vi "Core-GetTicks.vi"(8 "error in (no error)":errorcluster, 11 "Engine in":refnum<class "Engine.lvclass">) -> (0 "error out":errorcluster, 3 "Engine out":refnum<class "Engine.lvclass">)   [LabVIEW 2024, in "GLF.lvlib" / "Engine.lvclass"]
uses:
  Engine.lvclass
  Engine.lvclass/Engine.ctl
  <vilib>/Saukko/LV SDL3/Sources/SDL3/Timer/Timer.lvlib
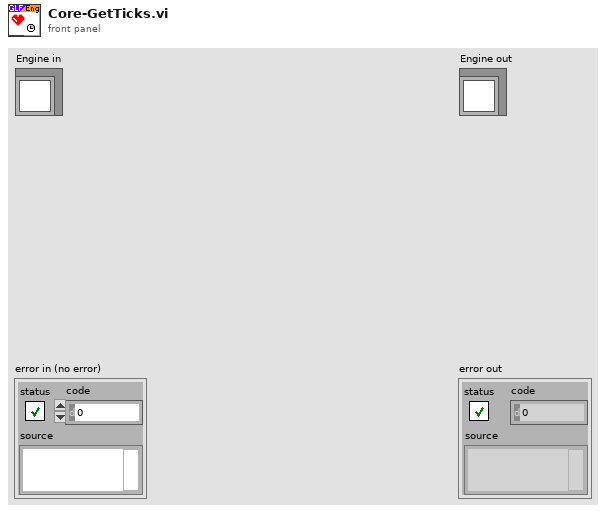
[diagram p1: front panel]
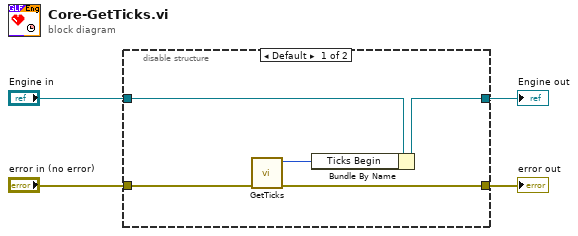
[diagram p0: block diagram]
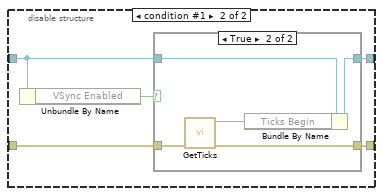
[diagram p2: hidden frame]
diagram:
  n1 = disable-structure shown="Default" {
    disable-tunnel: "error in (no error)" -> [w9 w14]
    disable-tunnel: "Engine in" -> [w8 w11]
    disable-tunnel: [w7 w13] -> w2
    disable-tunnel: [w5 w12] -> w1
    frame condition #0 (active) {
      n2 = call <vilib>:"GetTicks.vi"("No Error"=w9) -> ("error out"=w5:errorcluster, "Ticks [ms]"=w6:u64)  [unwired: 9 in]
      n3 = Bundle By Name(cluster=w8, "Ticks Begin"=w6) -> (w7:refnum<class "Engine.lvclass">)
    }
    frame condition #1 {
      n4 = Unbundle By Name(w11) -> ("VSync Enabled"=w10:bool)
      n5 = case shown="True" w10 {
        tunnel: w14 -> [w15 w21]
        tunnel: w11 -> [w16 w20]
        tunnel: [w16 w19] -> w13
        tunnel: [w15 w17] -> w12
        frame False {
        }
        frame True {
          n6 = call <vilib>:"GetTicks.vi"("No Error"=w21) -> ("error out"=w17:errorcluster, "Ticks [ms]"=w18:u64)  [unwired: 9 in]
          n7 = Bundle By Name(cluster=w20, "Ticks Begin"=w18) -> (w19:refnum<class "Engine.lvclass">)
        }
      }
    }
  }
  "error out" <- w1
  "Engine out" <- w2
